vi "UIOutputFGV.vi"(8 "FGVAction (Read)":T1, 11 "UIOutputIn":T2) -> (2 "Updated?":bool, 3 "UIOutputOut":T2)   [LabVIEW 2019]
uses:
  UIOutput.ctl
  UIOutputFGVAction.ctl
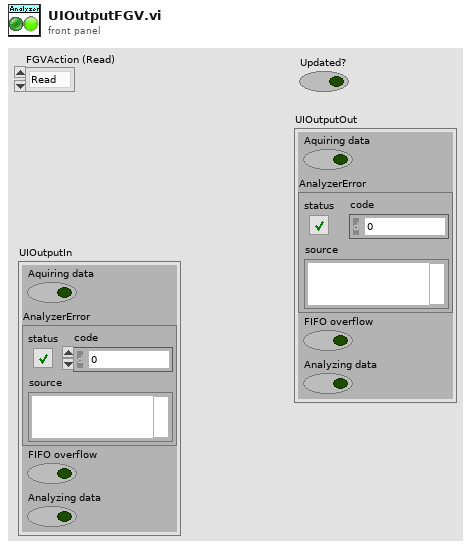
[diagram p1: front panel]
types:
  T1 = typedef "UIOutputFGVAction.ctl" = enum16{"Read", "Write", "CheckUpdate", "SetUpdated"}
  T2 = typedef "UIOutput.ctl" = cluster{"Aquiring data":bool, "AnalyzerError":errorcluster, "FIFO overflow":bool, "Analyzing data":bool}
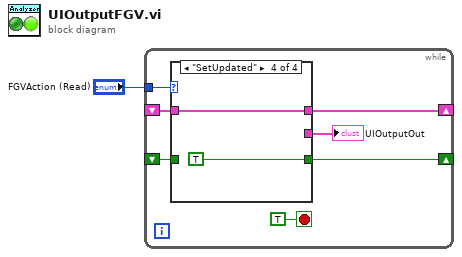
[diagram p0: block diagram]
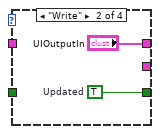
[diagram p3: hidden frame]
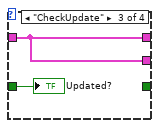
[diagram p4: hidden frame]
diagram:
  n1 = while {
    tunnel: "FGVAction (Read)" -> [w7]
    shift-right: [w5] -> _
    shift-left: _ -> [w6]
    shift-right: [w4] -> _
    shift-left: _ -> [w3]
    stop <- TRUE stop-if-true
    n2 = case shown="\"SetUpdated\"" w7 {
      tunnel: w6 -> [w9 _ w14 w16]
      tunnel: [w9 "UIOutputIn" w14 w16] -> w5
      tunnel: [w10 w11 _ TRUE ("Updated")] -> w4
      tunnel: w3 -> [w10 _ w13 _]
      tunnel: [w9 _ w14 _] -> w2
      frame "Read", Default {
      }
      frame "Write" {
        w11 = TRUE  # Updated
      }
      frame "CheckUpdate" {
        "Updated?" <- w13
      }
      frame "SetUpdated" {
      }
    }
    "UIOutputOut" <- w2
  }
